vi "QR Code_Detect QR Code.vi"(8 "error in":errorcluster, 10 "ROI Descriptor":T1 {"Contours"."Type" items=["No Selection", "Point", "Line", "Rectangle", "Oval", "Polygon", "Freehand Region", "Annulus", "Unused2", "Unused3", "Broken Line", "Freehand Line", "Rotated Rectangle"]}, 11 "Buffer Data In":T9) -> (0 "error out":errorcluster, 2 "QR Code Report":T2={"Found?"=FALSE, "Data"="", "Bounding Box"=[], "Errors Corrected"=0, "Dimensions (Rows/Cols)"=0, "Version"=0, "QR Model"=0, "Stream Mode"=0, "Barcode Polarity"=-2, "Mirrored?"=FALSE, "Append Stream Position"=0, "Size of Append Stream"=0, "First EAN-128 ID"=0, "First Alternate Language ID"=0, "Append Stream ID"=0, "Minimum Edge Strength"=30, "Demodulation Mode"=-2, "Cell Sample Size"=-2, "Cell Filter Mode"=-2} {"Append Stream ID" format="%x"; "Cell Filter Mode" items=["Auto-detect"=-2, "Average"=0, "Median"=1, "Central Average"=2, "High Average"=3, "Low Average"=4, "Very High Average"=5, "Very Low Average"=6, "All Filters"=8]; "Cell Sample Size" items=["Auto-detect"=-2, "1x1"=1, "2x2"=2, "3x3"=3, "4x4"=4, "5x5"=5, "6x6"=6, "7x7"=7]; "Demodulation Mode" items=["Auto-detect"=-2, "Histogram"=0, "Local Contrast"=1, "Combination"=2, "All"=3]; "Barcode Polarity" items=["Auto-detect"=-2, "Black on White"=0, "White on Black"=1]; "Stream Mode" items=["Numeric", "AlphaNumeric", "Raw Bytes", "UCC/EAN-128 - In Tokens", "UCC/EAN-128 - In Data", "Extended Character Interpretation", "Kanji"]; "QR Model" items=["Auto-detect", "Micro", "Model 1", "Model 2"]; "Version" max=40 step=1}, 3 "Buffer Data Out":T9)   [LabVIEW 2016]
uses:
  Data Def/QR Code_Buffer Data.ctl
  <vilib>/vision/Image Controls.llb/IMAQ Image.ctl
  <vilib>/vision/Instrument.llb/QR Code Report.ctl
  <vilib>/vision/Instrument.llb/QR Code Model Type.ctl
  <vilib>/vision/Instrument.llb/QR Code Stream Mode Type.ctl
  <vilib>/vision/Instrument.llb/Data Matrix Polarity.ctl
  <vilib>/vision/Instrument.llb/Demodulation Mode.ctl
  <vilib>/vision/Instrument.llb/Cell Sample Size.ctl
  <vilib>/vision/Instrument.llb/Cell Filter Mode.ctl
  <vilib>/vision/NI_Vision_Development_Module.lvlib
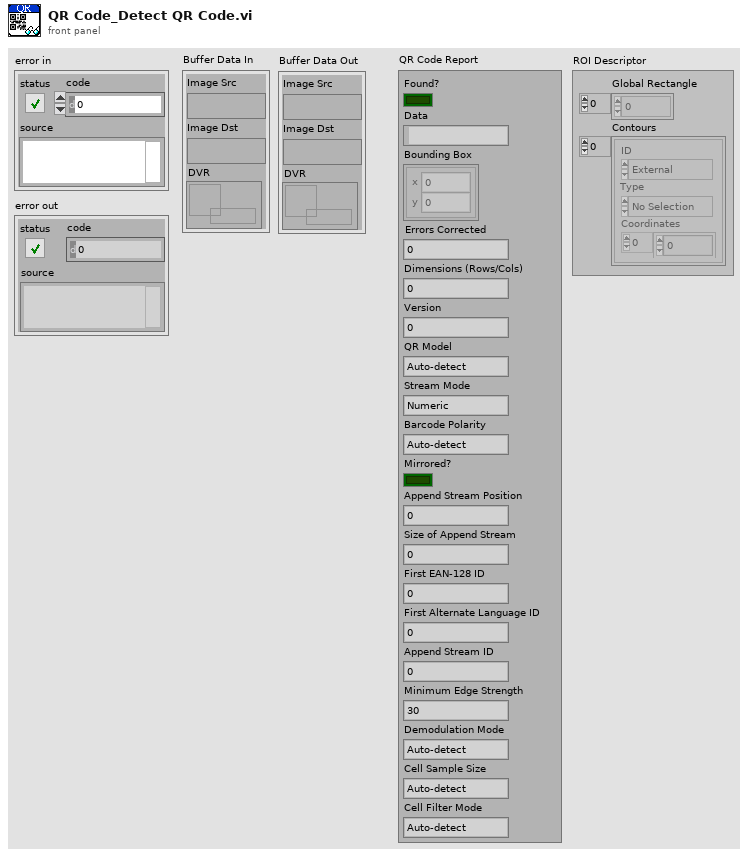
[diagram p1: front panel]
types:
  T1 = typedef "ROI Descriptor" = cluster{"Global Rectangle":i32[], "Contours":cluster{"ID":enum32{"External", "Internal"}, "Type":u32, "Coordinates":i32[]}[]}
  T2 = typedef "QR Code Report.ctl" = cluster{"Found?":bool, "Data":string, "Bounding Box":cluster{"x":sgl, "y":sgl}[], "Errors Corrected":u32, "Dimensions (Rows/Cols)":u32, "Version":u32, "QR Model":T3, "Stream Mode":T4, "Barcode Polarity":T5, "Mirrored?":bool, "Append Stream Position":u32, "Size of Append Stream":u32, "First EAN-128 ID":i32, "First Alternate Language ID":i32, "Append Stream ID":u32, "Minimum Edge Strength":u32, "Demodulation Mode":T6, "Cell Sample Size":T7, "Cell Filter Mode":T8}
  T3 = typedef "QR Code Model Type.ctl" = i32
  T4 = typedef "QR Code Stream Mode Type.ctl" = i32
  T5 = typedef "Data Matrix Polarity.ctl" = i32
  T6 = typedef "Demodulation Mode.ctl" = i32
  T7 = typedef "Cell Sample Size.ctl" = i32
  T8 = typedef "Cell Filter Mode.ctl" = i32
  T9 = typedef "QR Code_Buffer Data.ctl" = cluster{"Image Src":T10, "Image Dst":T10, "DVR":refnum<data-value>}
  T10 = typedef "IMAQ Image.ctl" = refnum<image>
  T11 = typedef "QR Code_QR Code Setting.ctl" = cluster{"QR Search Options":T12, "QR Description Options":T13, "QR Code Cell Size (pixels)":cluster{"Minimum Size":u32, "Maximum Size":u32}}
  T12 = typedef "QR Code Search Options.ctl" = cluster{"Rotation Mode":enum32{"Unlimited", "0 Degrees", "90 Degrees", "180 Degrees", "270 Degrees"}, "Skip Location?":bool, "Edge Threshold":u32, "Demodulation Mode":T6, "Cell Sample Size":T7, "Cell Filter Mode":T8, "Skew Degrees Allowed":u32}
  T13 = typedef "QR Code Description Options.ctl" = cluster{"Matrix Size (cells)":i32, "Barcode Polarity":T5, "Mirror Mode":i32, "QR Model":T3}
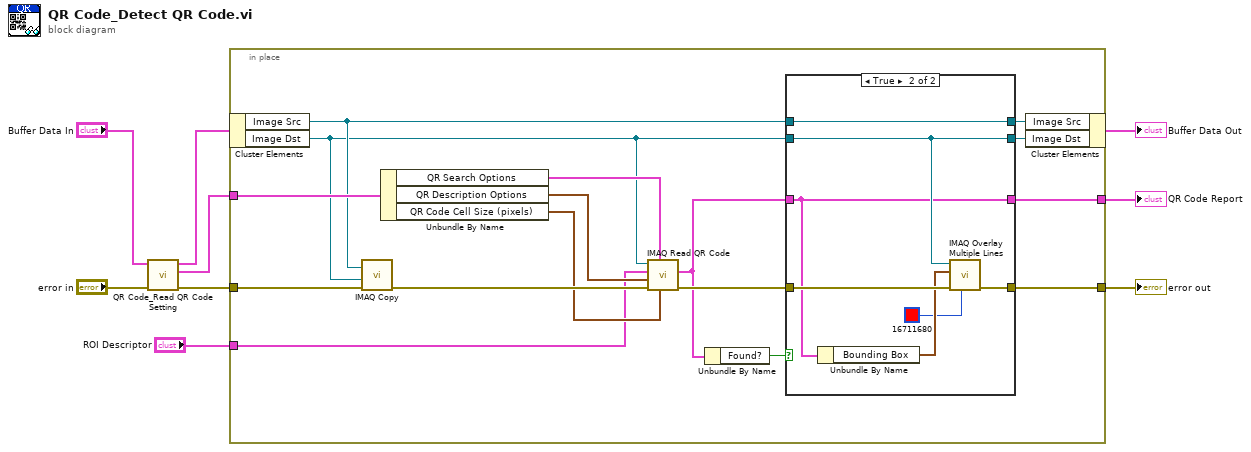
[diagram p0: block diagram]
diagram:
  n1 = call "QR Code_Read QR Code Setting.vi"("error in"="error in", "Buffer Data In"="Buffer Data In") -> ("error out"=w6:errorcluster, "QR Code Setting"=w5:T11, "Buffer Data Out"=w7:T9)  [unwired: 7 in]
  n2 = in-place {
    in-place-border: w6 -> [w25]
    in-place-border: w5 -> [w23]
    in-place-border: [w12] -> w3
    in-place-border: [w11] -> w2
    in-place-border: "ROI Descriptor" -> [w10]
    n3 = in-place-cluster #1(w7) -> ("Image Src"=w18:T10, "Image Dst"=w17:T10)
    n4 = call "IMAQ Copy"("error in (no error)"=w25, "Image Dst"=w17, "Image Src"=w18) -> ("error out"=w24:errorcluster)  [unwired: 3 in, 1 out]
    n5 = Unbundle By Name(w23) -> ("QR Search Options"=w22:T12, "QR Description Options"=w21:T13, "QR Code Cell Size (pixels)"=w20:cluster{"Minimum Size":u32, "Maximum Size":u32})
    n6 = call "IMAQ Read QR Code"("QR Code Cell Size (pixels)"=w20, "QR Search Options"=w22, "error in (no error)"=w24, "QR Description Options"=w21, "ROI Descriptor"=w10, "Image"=w17) -> ("error out"=w14:errorcluster, "QR Code Report"=w13:T2)  [unwired: 2 in, 2 out]
    n7 = Unbundle By Name(w13) -> ("Found?"=w19:bool)
    n8 = case shown="True" w19 {
      tunnel: w18 -> [w26 w34]
      tunnel: w17 -> [w27 w33]
      tunnel: [w26 w34] -> w16
      tunnel: [w27 w33] -> w15
      tunnel: w14 -> [w29 w36]
      tunnel: w13 -> [w28 w30]
      tunnel: [w29 w31] -> w12
      tunnel: [w28 w30] -> w11
      frame False {
      }
      frame True {
        n9 = Unbundle By Name(w30) -> ("Bounding Box"=w35:cluster{"x":sgl, "y":sgl}[])
        n10 = call "IMAQ Overlay Multiple Lines"("Color"=u32 16711680, "error in (no error)"=w36, "Line End Points"=w35, "Image"=w33) -> ("error out"=w31:errorcluster)  [unwired: 6 in, 1 out]
      }
    }
    n11 = in-place-cluster #1("Image Src"=w16, "Image Dst"=w15) -> (→"Buffer Data Out":T9)
  }
  "error out" <- w3
  "QR Code Report" <- w2
